vi "Register.vi"(8 "error in (no error)":errorcluster, 11 "Web FP In":refnum<class "Web Front Panel.lvclass">) -> (0 "error out":errorcluster, 2 "Created JS":path, 3 "Created HTML":path)   [LabVIEW 2015, in "Front Panel Publisher.lvlib" / "Front Panel Manager.lvclass"]
doc: "Register another WebFrontPanel"
uses:
  Front Panel Manager.lvclass
  Web Front Panel_class/Web Front Panel.lvclass
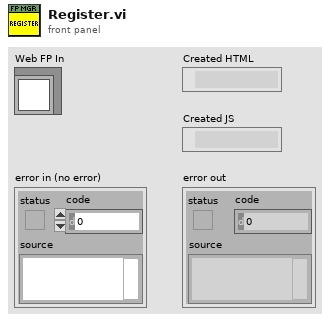
[diagram p1: front panel]
types:
  T1 = typedef "Front Panel Publisher.lvlib/Front Panel Manager.lvclass/Object Attributes.ctl" = cluster{"WebFrontPanels":refnum<class "Web Front Panel.lvclass">[], "WFP Names":string[], "Root folder":path, "Websocket Info":T2}
  T2 = typedef "Front Panel Publisher.lvlib/Front Panel Manager.lvclass/Websocket Info.ctl" = cluster{"Hostname":string, "Port":u16}
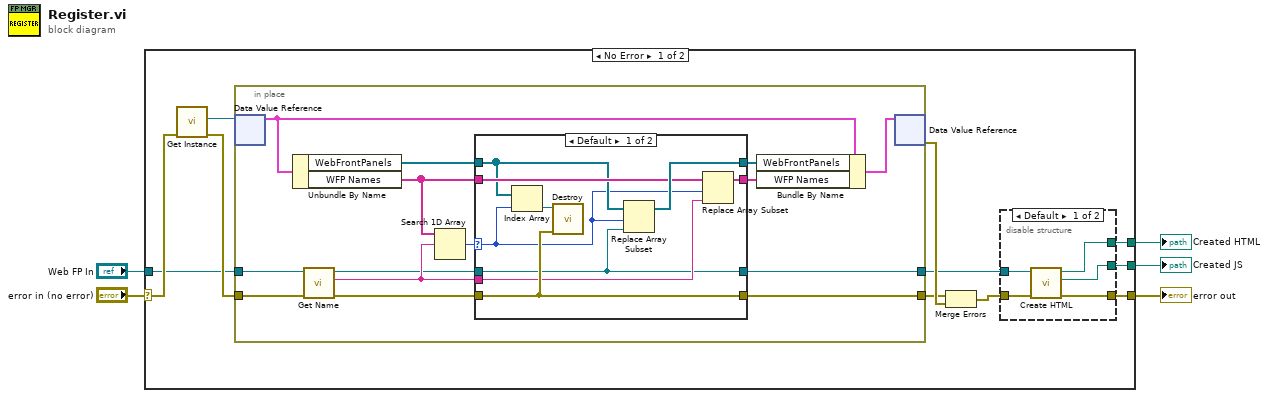
[diagram p0: block diagram]
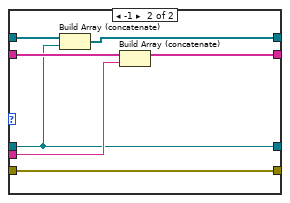
[diagram p3: hidden frame]
diagram:
  n1 = case shown="No Error" "error in (no error)" {
    selector: "error in (no error)" -> [w15 w53]
    tunnel: [w11 w53] -> w4
    tunnel: "Web FP In" -> [w9 _]
    tunnel: [w7 _] -> w2
    tunnel: [w6 _] -> w1
    frame No Error {
      n2 = call "Get Instance.vi"("error in (no error)"=w15) -> ("error out"=w14:errorcluster, "DVRRefOut"=w10:refnum<data-value>)  [unwired: 6 in, 3 out]
      n3 = in-place {
        in-place-border: w9 -> [w30]
        in-place-border: w14 -> [w36]
        in-place-border: [w35] -> w13
        in-place-border: [w23] -> w8
        n4 = in-place-dvr #1(w10) -> (w27:T1)  [unwired: 1 out]
        n5 = Unbundle By Name(w27) -> ("WebFrontPanels"=w33:refnum<class "Web Front Panel.lvclass">[], "WFP Names"=w29:string[])
        n6 = call-dynamic "Get Name.vi"("error in (no error)"=w36, "Web FP In"=w30) -> ("error out"=w34:errorcluster, "WFP Name"=w25:string, "Web FP Out"=w24:refnum<class "Web Front Panel.lvclass">)  [unwired: 7 in]
        n7 = Search 1D Array(1D array=w29, element=w25) -> (index of element=w31:i32)  [unwired: 1 in]
        n8 = case shown="Default" w31 {
          selector: w31 -> [w39 _]
          tunnel: w33 -> [w40 w51]
          tunnel: w24 -> [w37 w46]
          tunnel: w29 -> [w43 w49]
          tunnel: [w44 w50] -> w32
          tunnel: [w42 w48] -> w28
          tunnel: w25 -> [w41 w47]
          tunnel: w34 -> [w45 w52]
          tunnel: [w45 w52] -> w35
          tunnel: [w37 w46] -> w23
          frame Default {
            n9 = Index Array(array=w40, index=w39) -> (element=w38:refnum<class "Web Front Panel.lvclass">)
            n10 = call-dynamic "Destroy.vi"("error in (no error)"=w45, "Web FP In"=w38) -> ()  [unwired: 8 in, 2 out]
            n11 = Replace Array Subset(array=w40, new element=w37, index=w39) -> (w44:refnum<class "Web Front Panel.lvclass">[])
            n12 = Replace Array Subset(array=w43, new element=w41, index=w39) -> (w42:string[])
          }
          frame -1 {
            n13 = Build Array (concatenate)(w51, w46) -> (w50:refnum<class "Web Front Panel.lvclass">[])
            n14 = Build Array (concatenate)(w49, w47) -> (w48:string[])
          }
        }
        n15 = Bundle By Name(cluster=w27, "WebFrontPanels"=w32, "WFP Names"=w28) -> (w26:T1)
        n16 = in-place-dvr #1(w26) -> (w16:errorcluster)  [unwired: 1 out]
      }
      n17 = Merge Errors(w13, w16) -> (w12:errorcluster)
      n18 = disable-structure shown="Default" {
        disable-tunnel: w12 -> [w21 w22]
        disable-tunnel: [w20 w22] -> w11
        disable-tunnel: w8 -> [w19 _]
        disable-tunnel: [w18 _] -> w7
        disable-tunnel: [w17 _] -> w6
        frame condition #0 (active) {
          n19 = call "Create HTML.vi"("error in (no error)"=w21, "Web FP In"=w19) -> ("error out"=w20:errorcluster, "Created JS"=w17:path, "Created HTML"=w18:path)  [unwired: 7 in]
        }
        frame condition #1 {
        }
      }
    }
    frame Error {
    }
  }
  "error out" <- w4
  "Created HTML" <- w2
  "Created JS" <- w1
